vi "Structures Demo.vi"   [LabVIEW 2020]
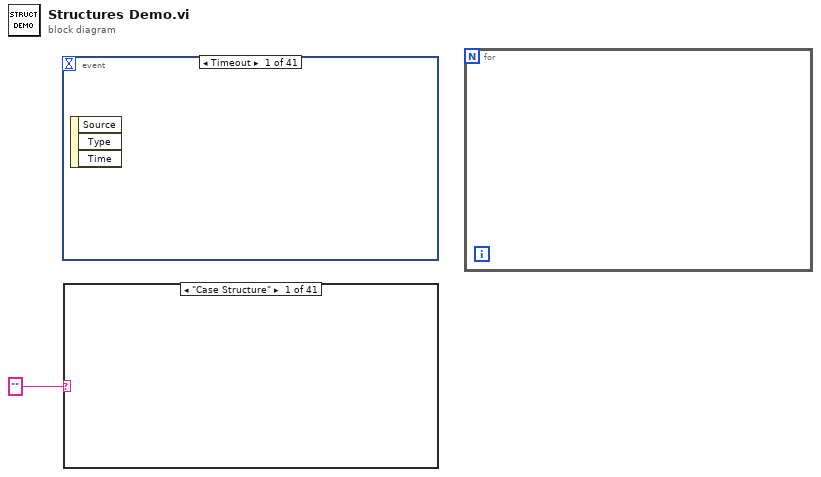
[diagram p0: block diagram]
diagram:
  n1 = event shown="[0] Timeout" {
    selector: _ -> [_ _ _ _ _ _ _ _ _ _ _ _ _ _ _ _ _ _ _ _ _ _ _ _ _ _ _ _ _ _ _ _ _ _ _ _ _ _ _ _ _]
    dyn-events: _ -> [_ _ _ _ _ _ _ _ _ _ _ _ _ _ _ _ _ _ _ _ _ _ _ _ _ _ _ _ _ _ _ _ _ _ _ _ _ _ _ _ _]
    timeout: _ -> [_ _ _ _ _ _ _ _ _ _ _ _ _ _ _ _ _ _ _ _ _ _ _ _ _ _ _ _ _ _ _ _ _ _ _ _ _ _ _ _ _]
    event Timeout {
      n2 = event-data() -> ()  [unwired: 1 in, 3 out]
    }
    event event #0x50 {
      n3 = event-data() -> ()  [unwired: 1 in, 3 out]
    }
    event event type 0.0.x8000004f {
      n4 = event-data() -> ()  [unwired: 1 in, 3 out]
      n5 = event-data() -> ()  [unwired: 2 in, 1 out]
    }
    event Application Instance Close {
      n6 = event-data() -> ()  [unwired: 1 in, 4 out]
    }
    event Application Instance Close? {
      n7 = event-data() -> ()  [unwired: 1 in, 5 out]
      n8 = event-data() -> ()  [unwired: 3 in, 1 out]
    }
    event Autoscale Range Change {
      n9 = event-data() -> ()  [unwired: 1 in, 3 out]
    }
    event event #0x52 {
      n10 = event-data() -> ()  [unwired: 1 in, 6 out]
    }
    event Edit Cell {
      n11 = event-data() -> ()  [unwired: 1 in, 3 out]
    }
    event event type 0.0.x80000037 {
      n12 = event-data() -> ()  [unwired: 1 in, 3 out]
      n13 = event-data() -> ()  [unwired: 2 in, 1 out]
    }
    event Cursor Grab {
      n14 = event-data() -> ()  [unwired: 1 in, 3 out]
    }
    event event type 0.0.x80000027 {
      n15 = event-data() -> ()  [unwired: 1 in, 3 out]
      n16 = event-data() -> ()  [unwired: 2 in, 1 out]
    }
    event event #0x4e {
      n17 = event-data() -> ()  [unwired: 1 in, 3 out]
    }
    event event type 0.0.x8000004d {
      n18 = event-data() -> ()  [unwired: 1 in, 3 out]
      n19 = event-data() -> ()  [unwired: 2 in, 1 out]
    }
    event Cursor Move {
      n20 = event-data() -> ()  [unwired: 1 in, 3 out]
    }
    event Cursor Release {
      n21 = event-data() -> ()  [unwired: 1 in, 3 out]
    }
    event Data Change {
      n22 = event-data() -> ()  [unwired: 1 in, 3 out]
    }
    event Direction Change {
      n23 = event-data() -> ()  [unwired: 1 in, 3 out]
    }
    event Display State Change {
      n24 = event-data() -> ()  [unwired: 1 in, 3 out]
    }
    event Drag Ended {
      n25 = event-data() -> ()  [unwired: 1 in, 3 out]
    }
    event event type 0.0.xa0000039 {
      n26 = event-data() -> ()  [unwired: 1 in, 3 out]
      n27 = event-data() -> ()  [unwired: 2 in, 1 out]
    }
    event event #0x3d {
      n28 = event-data() -> ()  [unwired: 1 in, 3 out]
    }
    event event type 0.0.xa000003a {
      n29 = event-data() -> ()  [unwired: 1 in, 3 out]
      n30 = event-data() -> ()  [unwired: 2 in, 1 out]
    }
    event event type 0.0.xa000002e {
      n31 = event-data() -> ()  [unwired: 1 in, 3 out]
      n32 = event-data() -> ()  [unwired: 2 in, 1 out]
    }
    event Drag Starting {
      n33 = event-data() -> ()  [unwired: 1 in, 3 out]
    }
    event event type 0.0.x8000002c {
      n34 = event-data() -> ()  [unwired: 1 in, 3 out]
      n35 = event-data() -> ()  [unwired: 2 in, 1 out]
    }
    event event type 0.0.xa000003e {
      n36 = event-data() -> ()  [unwired: 1 in, 3 out]
      n37 = event-data() -> ()  [unwired: 2 in, 1 out]
    }
    event Exec State Change {
      n38 = event-data() -> ()  [unwired: 1 in, 3 out]
    }
    event Key Down {
      n39 = event-data() -> ()  [unwired: 1 in, 8 out]
    }
    event Key Down? {
      n40 = event-data() -> ()  [unwired: 1 in, 8 out]
      n41 = event-data() -> ()  [unwired: 6 in, 1 out]
    }
    event Key Repeat {
      n42 = event-data() -> ()  [unwired: 1 in, 8 out]
    }
    event event type 5.0.x8000000b {
      n43 = event-data() -> ()  [unwired: 1 in, 8 out]
      n44 = event-data() -> ()  [unwired: 6 in, 1 out]
    }
    event Key Up {
      n45 = event-data() -> ()  [unwired: 1 in, 8 out]
    }
    event Double Click {
      n46 = event-data() -> ()  [unwired: 1 in, 3 out]
    }
    event event type 0.0.x80000020 {
      n47 = event-data() -> ()  [unwired: 1 in, 3 out]
      n48 = event-data() -> ()  [unwired: 2 in, 1 out]
    }
    event Menu Selection (App) {
      n49 = event-data() -> ()  [unwired: 1 in, 7 out]
    }
    event Menu Selection? (App) {
      n50 = event-data() -> ()  [unwired: 1 in, 7 out]
      n51 = event-data() -> ()  [unwired: 2 in, 1 out]
    }
    event Menu Selection (User) {
      n52 = event-data() -> ()  [unwired: 1 in, 7 out]
    }
    event Mouse Down {
      n53 = event-data() -> ()  [unwired: 1 in, 3 out]
    }
    event event type 0.0.x80000007 {
      n54 = event-data() -> ()  [unwired: 1 in, 3 out]
      n55 = event-data() -> ()  [unwired: 2 in, 1 out]
    }
    event Mouse Enter {
      n56 = event-data() -> ()  [unwired: 1 in, 4 out]
    }
    event #40 (no event record) {
      n57 = event-data() -> ()  [unwired: 1 in, 3 out]
    }
  }
  n58 = case shown="\"Case Structure\"" "" {
    frame "Case Structure" {
    }
    frame "0" {
    }
    frame "1" {
    }
    frame "2" {
    }
    frame "3" {
    }
    frame "4" {
    }
    frame "5" {
    }
    frame "6" {
    }
    frame "7" {
    }
    frame "8" {
    }
    frame "9" {
    }
    frame "10" {
    }
    frame "11" {
    }
    frame "12" {
    }
    frame "13" {
    }
    frame "14" {
    }
    frame "15" {
    }
    frame "16" {
    }
    frame "17" {
    }
    frame "18" {
    }
    frame "19" {
    }
    frame "20" {
    }
    frame "21" {
    }
    frame "22" {
    }
    frame "23" {
    }
    frame "24" {
    }
    frame "25" {
    }
    frame "26" {
    }
    frame "27" {
    }
    frame "28" {
    }
    frame "29" {
    }
    frame "30" {
    }
    frame "31" {
    }
    frame "32" {
    }
    frame "33" {
    }
    frame "34" {
    }
    frame "35" {
    }
    frame "36" {
    }
    frame "37" {
    }
    frame "38" {
    }
    frame "39" {
    }
  }
  n59 = for {
  }
